vi "Configure Aperture.vi"(8 "error in (no error)":errorcluster, 9 "Aperture Time (0.1 seconds)":dbl(ring)=0.1 items=["0.01"=0.01, "0.1"=0.1, "1.0"=1.0], 10 "Function (6: Frequency)":u16(ring)=6 items=["DC Voltage", "AC Voltage", "2 - Wire Resistance", "4 - Wire Resistance", "DC Current", "AC Current", "Frequency", "Period", "Continuity", "Diode Checking", "Temperature", "Capacitance"], 11 "VISA resource name":refnum<visa-resource-name>) -> (0 "error out":errorcluster, 3 "VISA resource name out":refnum<visa-resource-name>)   [LabVIEW 2010, in "Fluke 884X Series.lvlib"]
doc: "Configures the Aperture Time for Frequency and Period measurement functions.\n\n<b>Note1:</b>\n Aperture Time is not applicable to the measurement functions below:\n AC/DC Voltage\n 2-Wire/4-Wire Resistance\n AC/DC Current\n Diode Checking\n Temperature\n Capacitance\n\n<B>Note2:</B>\n\nFluke 8845A does not support Temperature or Capacitance configurations or measurements."
uses:
  <instrlib>/Fluke 884X Series/Fluke 884X Series.lvlib
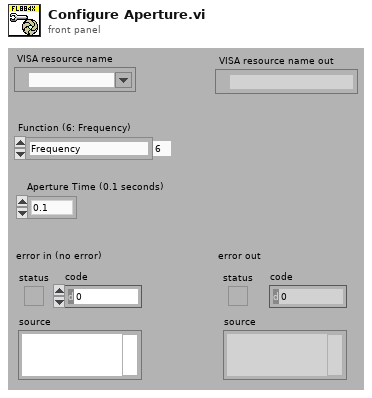
[diagram p1: front panel]
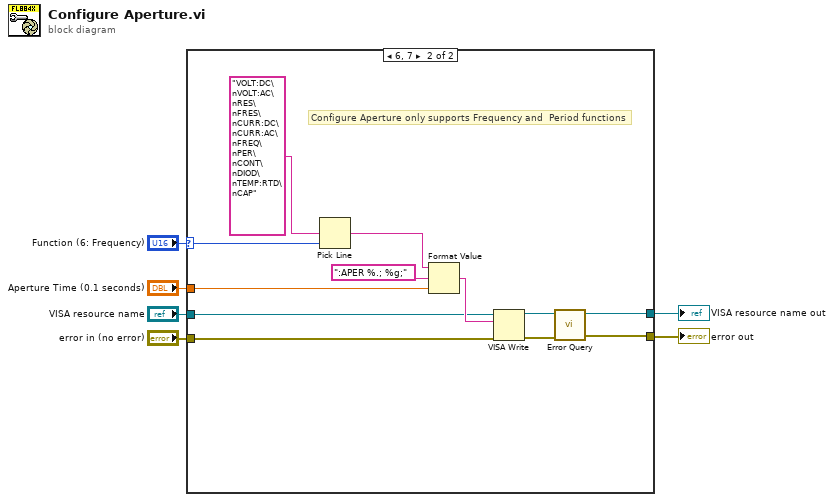
[diagram p0: block diagram]
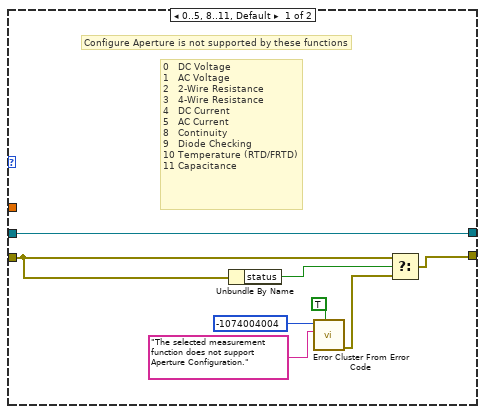
[diagram p2: hidden frame]
diagram:
  n1 = case shown="6, 7" "Function (6: Frequency)" {
    selector: "Function (6: Frequency)" -> [_ w20]
    tunnel: "VISA resource name" -> [w14 w18]
    tunnel: "error in (no error)" -> [w9 w17]
    tunnel: [w7 w24] -> w3
    tunnel: [w14 w23] -> w2
    tunnel: "Aperture Time (0.1 seconds)" -> [_ w15]
    frame 0..5, 8..11, Default {
      # "Configure Aperture is not supported by these functions"
      # "0   DC Voltage\n1   AC Voltage\n2   2-Wire Resistance\n3   4-Wire Resistance\n4   DC Current\n5   AC Current\n8   Continuity\n9   Diode Checking\n10 Temperature (RTD/FRTD)\n11 Capacitance"
      n2 = Unbundle By Name(w9) -> ("status"=w10:bool)
      n3 = call <vilib>:"Error Cluster From Error Code.vi"("show call chain? (False)"=TRUE, "error message (\"\")"="The selected measurement function does not support Aperture Configuration." ("Source (VI Name)"), "error code (0)"=-1074004004 ("Code")) -> ("error out"=w8:errorcluster)  [unwired: 6 in]
      n4 = Select(t=w9, s=w10, f=w8) -> (s? t:f=w7:errorcluster)
    }
    frame 6, 7 {
      # "Configure Aperture only supports Frequency and  Period functions"
      n5 = Pick Line(multi-line string="VOLT:DC\nVOLT:AC\nRES\nFRES\nCURR:DC\nCURR:AC\nFREQ\nPER\nCONT\nDIOD\nTEMP:RTD\nCAP", line index=w20) -> (output string=w19:string)  [unwired: 1 in]
      n6 = Format Value(string ("")=w19, format string=":APER %.; %g;", value (0)=w15) -> (output string=w21:string)
      n7 = VISA Write(VISA resource name=w18, write buffer=w21, error in (no error)=w17) -> (VISA resource name out=w26:refnum<visa-resource-name>, error out=w25:errorcluster)  [unwired: 1 out]
      n8 = call <instrlib>:"Error Query.vi"("error in (no error)"=w25, "VISA resource name"=w26) -> ("error out"=w24:errorcluster, "VISA resource name out"=w23:refnum<visa-resource-name>)  [unwired: 6 in, 2 out]
    }
  }
  "error out" <- w3
  "VISA resource name out" <- w2
